vi "tune result to pp string.vi"(8 "error in (no error)":errorcluster, 9 "strbuffer_len":u64, 10 "pp_string_out":string, 11 "tune_result":T1) -> (0 "error out":errorcluster, 2 "pp_string_out out":string, 3 "tune_result out":T1)   [LabVIEW 2023, in "uhd.lvlib"]
doc: "UHD_API void uhd_tune_result_to_pp_string(\n uhd_tune_result_t* tune_result, char* pp_string_out, size_t strbuffer_len);"
uses:
  <userlib>/uhd/uhd.lvlib
  <userlib>/uhd/uhd.dll
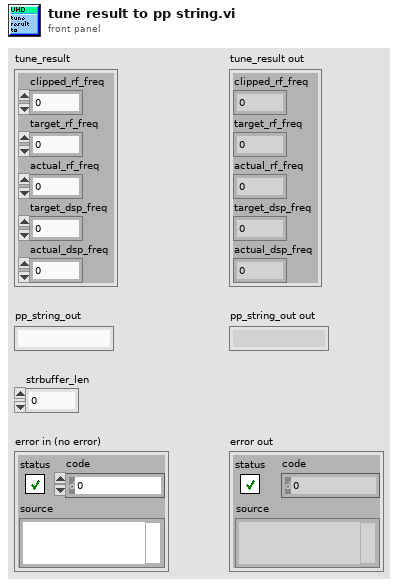
[diagram p1: front panel]
types:
  T1 = cluster{"clipped_rf_freq":dbl, "target_rf_freq":dbl, "actual_rf_freq":dbl, "target_dsp_freq":dbl, "actual_dsp_freq":dbl}
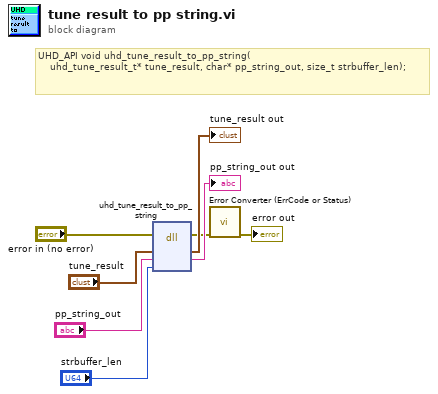
[diagram p0: block diagram]
diagram:
  # "UHD_API void uhd_tune_result_to_pp_string(\n    uhd_tune_result_t* tune_result, char* pp_string_out, size_t strbuffer_len);"
  n1 = dll-call lib="C:/Program Files/National Instruments/LabVIEW 2023/user.lib/uhd/uhd.*" fn="uhd_tune_result_to_pp_string"(error in="error in (no error)", "tune_result"="tune_result", "pp_string_out"="pp_string_out", "strbuffer_len"="strbuffer_len") -> (error out=w2:errorcluster, "tune_result"=→"tune_result out":T1, "pp_string_out"=→"pp_string_out out":string)  [unwired: 4 in, 1 out]
  n2 = call <userlib>:"Error Converter (ErrCode or Status).vi"("error in (no error)"=w2) -> ("error out"=→"error out":errorcluster)  [unwired: 10 in]
